vi "Handle Specific DAQ Errors.vi"(8 "error in (no error)":errorcluster, 10 "Error In":string, 11 "code":i32) -> (0 "error out":errorcluster, 3 "Error Message":string, 5 "Alert User?":bool)   [LabVIEW 2015]
doc: "This VI implements a moving average filter for this particular channel"
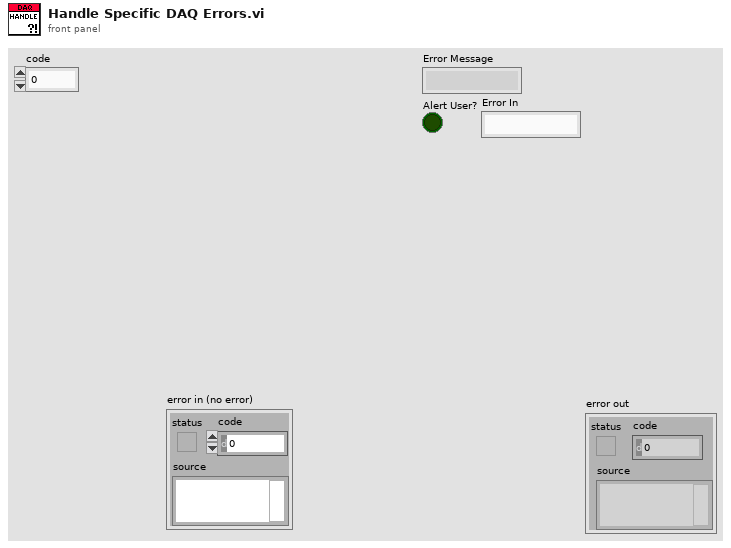
[diagram p1: front panel]
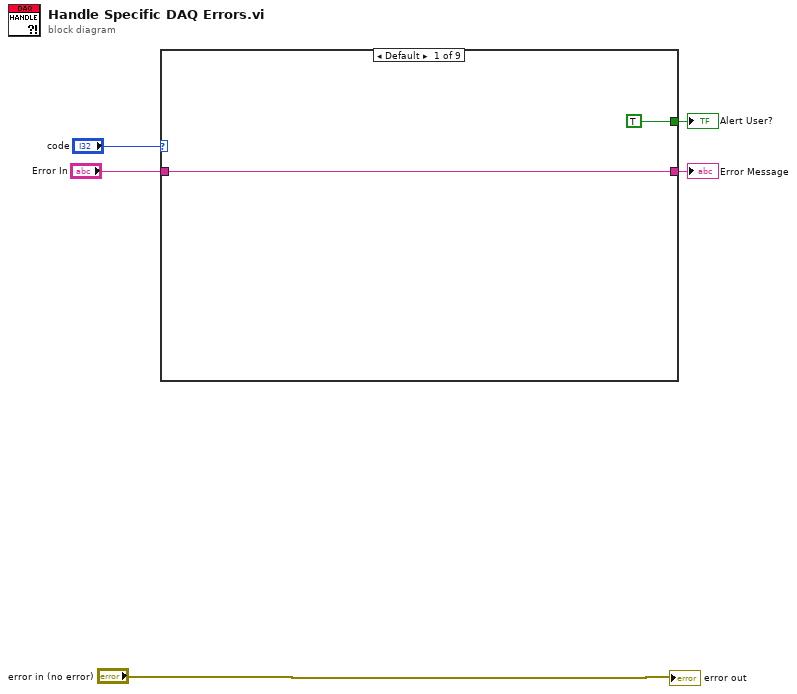
[diagram p0: block diagram]
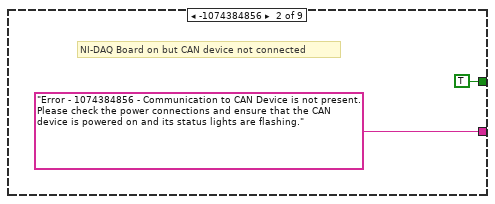
[diagram p2: hidden frame]
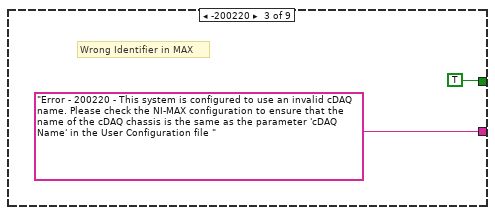
[diagram p3: hidden frame]
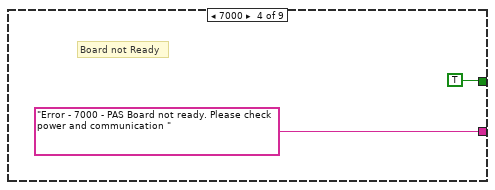
[diagram p4: hidden frame]
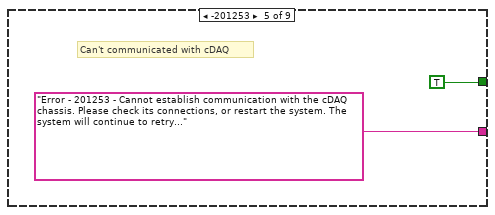
[diagram p5: hidden frame]
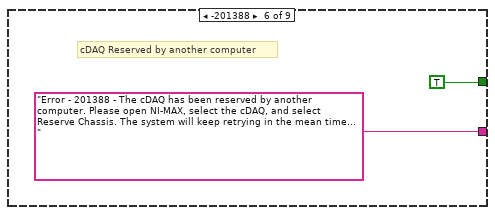
[diagram p6: hidden frame]
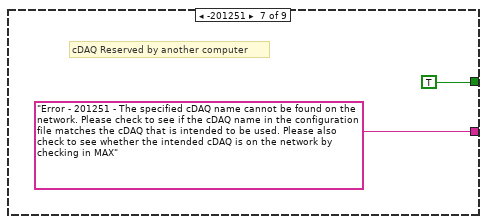
[diagram p7: hidden frame]
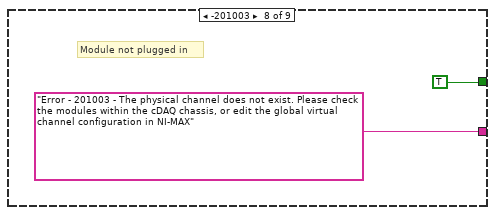
[diagram p8: hidden frame]
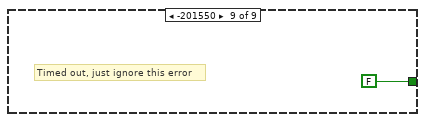
[diagram p9: hidden frame]
diagram:
  n1 = case shown="Default" "code" {
    tunnel: [w6 "Error - 1074384856 - Communication to CAN Device is not present. Please check the power connections and ensure that the CAN device is powered on and its status lights are flashing." "Error - 200220 - This system is configured to use an invalid cDAQ name. Please check the NI-MAX configuration to ensure that the name of the cDAQ chassis is the same as the parameter 'cDAQ Name' in the User Configuration file " "Error - 7000 - PAS Board not ready. Please check power and communication " "Error - 201253 - Cannot establish communication with the cDAQ chassis. Please check its connections, or restart the system. The system will continue to retry..." "Error - 201388 - The cDAQ has been reserved by another computer. Please open NI-MAX, select the cDAQ, and select Reserve Chassis. The system will keep retrying in the mean time... " "Error - 201251 - The specified cDAQ name cannot be found on the network. Please check to see if the cDAQ name in the configuration file matches the cDAQ that is intended to be used. Please also check to see whether the intended cDAQ is on the network by checking in MAX" "Error - 201003 - The physical channel does not exist. Please check the modules within the cDAQ chassis, or edit the global virtual channel configuration in NI-MAX" _] -> w3
    tunnel: [TRUE TRUE TRUE TRUE TRUE TRUE TRUE TRUE FALSE] -> w2
    tunnel: "Error In" -> [w6 _ _ _ _ _ _ _ _]
    frame Default {
    }
    frame -1074384856 {
      # "NI-DAQ Board on but CAN device not connected"
    }
    frame -200220 {
      # "Wrong Identifier in MAX"
    }
    frame 7000 {
      # "Board not Ready"
    }
    frame -201253 {
      # "Can't communicated with cDAQ"
    }
    frame -201388 {
      # "cDAQ Reserved by another computer"
    }
    frame -201251 {
      # "cDAQ Reserved by another computer"
    }
    frame -201003 {
      # "Module not plugged in"
    }
    frame -201550 {
      # "Timed out, just ignore this error"
    }
  }
  "Error Message" <- w3
  "Alert User?" <- w2
  "error out" <- "error in (no error)"
